vi "LVClass_Camera Read Image.vi"(8 "error in (no error)":errorcluster, 11 "Camera in":refnum<class "Camera.lvclass">) -> (0 "error out":errorcluster, 2 "Image.lvclass":refnum<class "Image.lvclass">, 3 "Camera out":refnum<class "Camera.lvclass">)   [LabVIEW 2020, in "Camera.lvclass"]
doc: "Get last captured image from camera object (internal image) \n\n<B>CameraIn</B> : Camera object.\n<B>CameraOut</B> : Camera object.\n<B>Image</B> : Captured image with (optionnally) background removed."
uses:
  Camera.lvclass
  Image/Image.lvclass
  Camera.lvclass/Camera.ctl
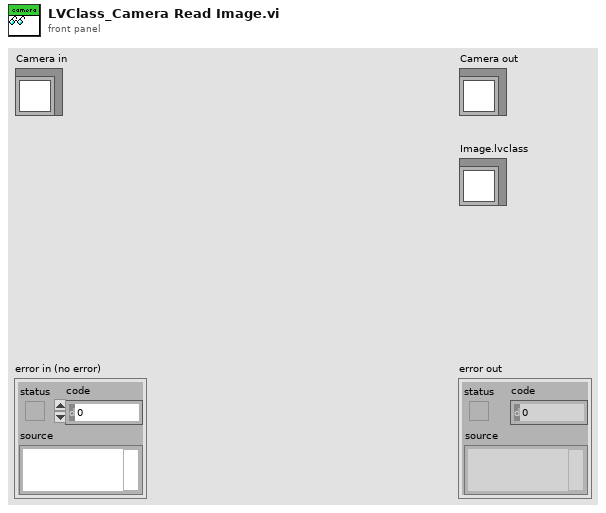
[diagram p1: front panel]
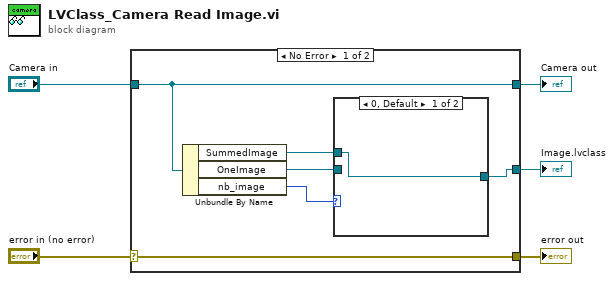
[diagram p0: block diagram]
diagram:
  n1 = case shown="No Error" "error in (no error)" {
    selector: "error in (no error)" -> [w11 w14]
    tunnel: [w11 w14] -> w4
    tunnel: [w10 w15] -> w2
    tunnel: "Camera in" -> [w10 w15]
    tunnel: [w7 _] -> w1
    frame No Error {
      n2 = Unbundle By Name(w10) -> ("SummedImage"=w9:refnum<class "Image.lvclass">, "OneImage"=w6:refnum<class "Image.lvclass">, "nb_image"=w8:u32)
      n3 = case shown="0, Default" w8 {
        tunnel: w9 -> [w12 _]
        tunnel: [w12 w13] -> w7
        tunnel: w6 -> [_ w13]
        frame 0, Default {
        }
        frame 1 {
        }
      }
    }
    frame Error {
    }
  }
  "error out" <- w4
  "Camera out" <- w2
  "Image.lvclass" <- w1
